vi "save_ref_data.vi"(6 "wl-current array":dbl[][](array[numeric]) caption="Data array", 8 "Pixel":string, 9 "Device label":string, 10 "Experiment Title":string, 11 "Username":string) -> (3 "Filepath out":path)   [LabVIEW 2016]
uses:
  <vilib>/Utility/file.llb/Write Delimited Spreadsheet (DBL).vi
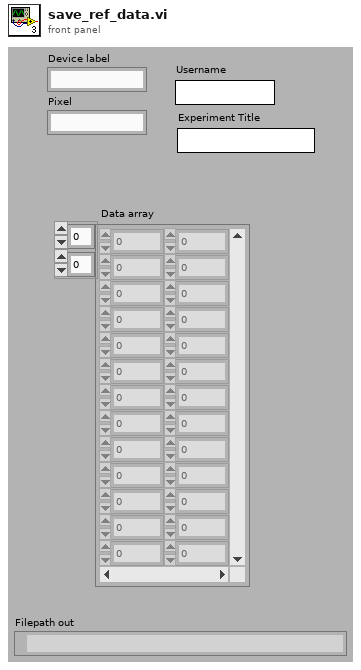
[diagram p1: front panel]
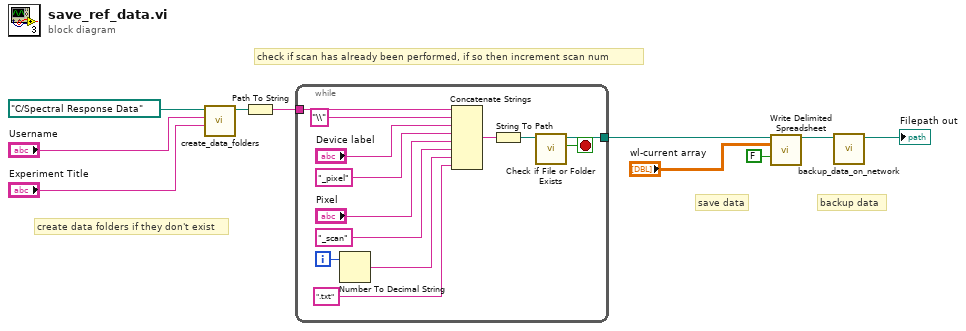
[diagram p0: block diagram]
diagram:
  # "backup data"
  # "save data"
  # "create data folders if they don't exist"
  # "check if scan has already been performed, if so then increment scan num"
  n1 = call "create_data_folders.vi"("Experiment Title"="Experiment Title", "Username"="Username", "Folderpath on C:"=path "C:/Spectral Response Data") -> ("Folderpath on C: out"=w9:path)  [unwired: 8 in]
  n2 = Path To String(path=w9) -> (string=w8:string)
  n3 = while {
    tunnel: [w12] -> w10
    tunnel: w8 -> [w23]
    i -> [w17]
    stop <- w11 stop-if-true
    n4 = Number To Decimal String(number=w17) -> (decimal integer string=w14:string)  [unwired: 1 in]
    n5 = Concatenate Strings(w23, "\\", "Device label", "_pixel", "Pixel", "_scan", w14, ".txt" ("string")) -> (w22:string)
    n6 = String To Path(string=w22) -> (path=w13:path)
    n7 = call <vilib>:"Check if File or Folder Exists.vi"("path"=w13) -> ("file or folder exists?"=w11:bool, "dup path"=w12:path)  [unwired: 8 in, 1 out]
  }
  n8 = call-poly <vilib>:"Write Delimited Spreadsheet.vi"("file path (dialog if empty)"=w10, "2D data"="wl-current array", "append to file? (new file:F)"=FALSE) -> ("new file path (Not A Path if cancelled)"=w4:path)  [unwired: 11 in, 1 out]
  n9 = call "backup_data_on_network.vi"("Filepath in"=w4) -> ("Filepath out"=→"Filepath out":path)  [unwired: 10 in]
